vi "Convolution by Real FFT.vi"(8 "error in (no error)":errorcluster, 10 "Array 2":dbl[](array[numeric]), 11 "Array 1":dbl[](array[numeric])) -> (0 "error out":errorcluster, 3 "Convolution":dbl[](array[numeric]))   [LabVIEW 2021, in "Math.lvlib"]
uses:
  <vilib>/Analysis/2dsp.llb/Real FFT.vi
  <vilib>/Analysis/2dsp.llb/Inverse Real FFT.vi
  <vilib>/Utility/error.llb/Error Cluster From Error Code.vi
  <vilib>/ErrorRing/Error Ring.xnode
  Math.lvlib
  <vilib>/Analysis/NI_AALPro.lvlib
  Error/Error.lvlib
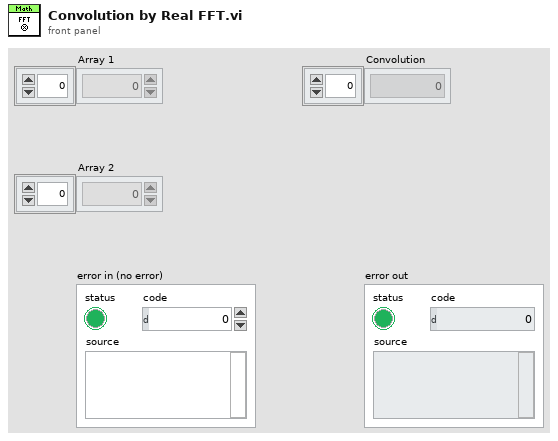
[diagram p1: front panel]
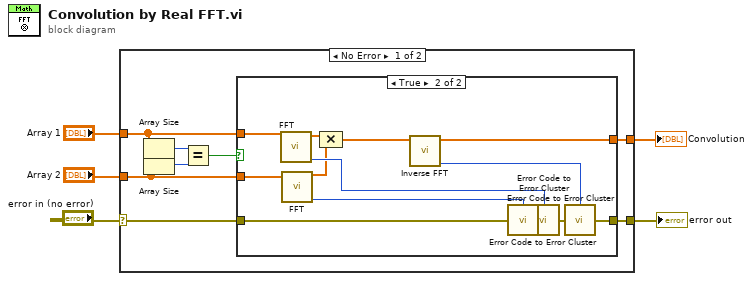
[diagram p0: block diagram]
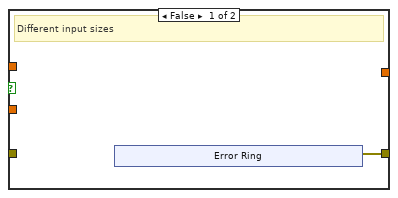
[diagram p2: hidden frame]
diagram:
  n1 = case shown="No Error" "error in (no error)" {
    selector: "error in (no error)" -> [w13 w32]
    tunnel: [w12 _] -> w4
    tunnel: [w11 w32] -> w3
    tunnel: "Array 1" -> [w10 _]
    tunnel: "Array 2" -> [w9 _]
    frame No Error {
      n2 = Array Size(array=w10) -> (size(s)=w8:i32)
      n3 = Array Size(array=w9) -> (size(s)=w7:i32)
      n4 = Equal?(x=w8, y=w7) -> (x = y?=w6:bool)
      n5 = case shown="True" w6 {
        tunnel: w13 -> [_ w31]
        tunnel: [_ w30] -> w12
        tunnel: [w14 w29] -> w11
        tunnel: w10 -> [_ w28]
        tunnel: w9 -> [_ w27]
        frame False {
          # "Different input sizes"
          n6 = xnode "Error Ring"() -> ("error out"=w14:errorcluster)
        }
        frame True {
          n7 = call-poly <vilib>:"FFT.vi"("X"=w28) -> ("error"=w25:i32, "FFT {X}"=w21:cdb[])  [unwired: 9 in]
          n8 = call-poly <vilib>:"FFT.vi"("X"=w27) -> ("error"=w26:i32, "FFT {X}"=w23:cdb[])  [unwired: 9 in]
          n9 = Compound Arithmetic op=MULTIPLY(w21, w23) -> (w22:cdb[])
          n10 = call-poly <vilib>:"Inverse FFT.vi"("FFT {X}"=w22) -> ("error"=w19:i32, "X"=w30:dbl[])  [unwired: 9 in]
          n11 = call "Error Code to Error Cluster.vi"("Error Code"=w26, "Error In"=w31) -> ("Error Out"=w24:errorcluster)  [unwired: 13 in]
          n12 = call "Error Code to Error Cluster.vi"("Error Code"=w25, "Error In"=w24) -> ("Error Out"=w20:errorcluster)  [unwired: 13 in]
          n13 = call "Error Code to Error Cluster.vi"("Error Code"=w19, "Error In"=w20) -> ("Error Out"=w29:errorcluster)  [unwired: 13 in]
        }
      }
    }
    frame Error {
    }
  }
  "error out" <- w3
  "Convolution" <- w4
